vi "Read data.vi"(7 "Command":T1, 8 "error in":errorcluster, 11 "file path":path) -> (0 "error out":errorcluster, 2 "Zone Setup Array":cluster{string, dbl}[](array[cluster]))   [LabVIEW 2013]
doc: "This SubVI is used to\n-Initialize the file path and stores it in shift register.\n-Reads the data from the stored file path.\n-Empty the file path."
uses:
  Controls/Read States.ctl
  <vilib>/Utility/file.llb/Read From Spreadsheet File (string).vi
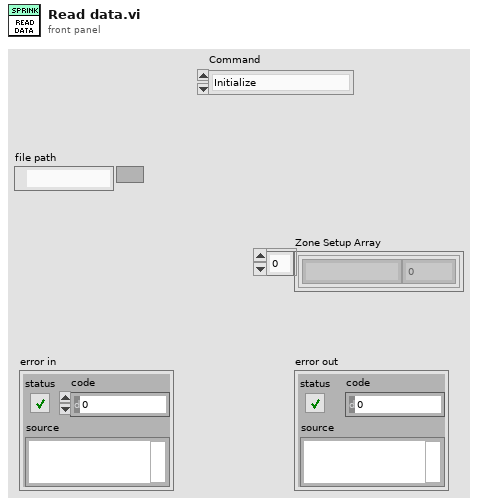
[diagram p1: front panel]
types:
  T1 = typedef "Read States.ctl" = enum16{"Initialize ", "Read", "Stop"}
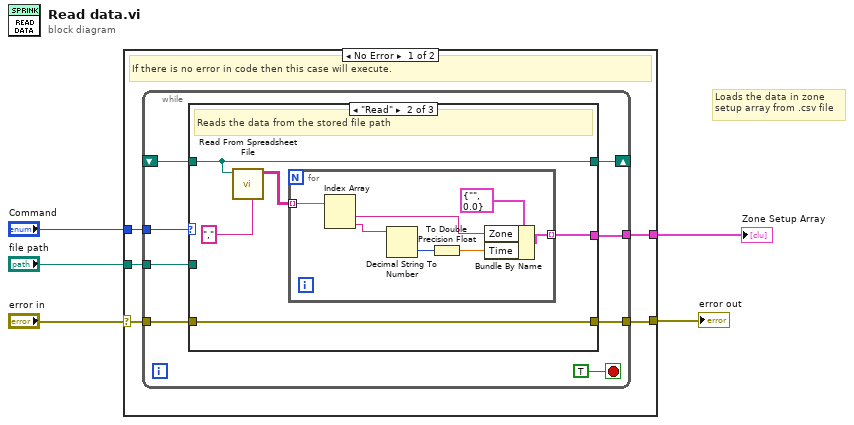
[diagram p0: block diagram]
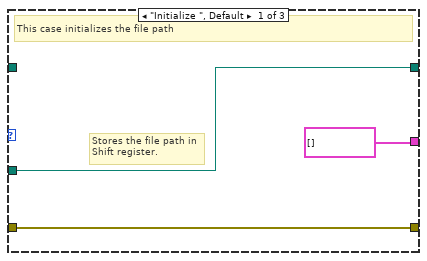
[diagram p2: hidden frame]
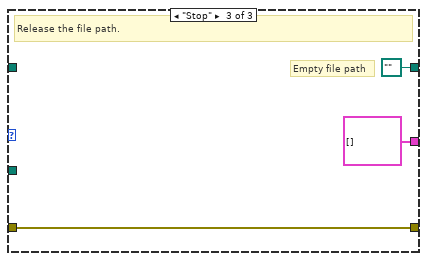
[diagram p3: hidden frame]
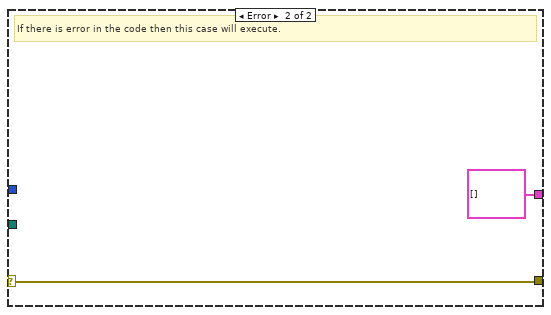
[diagram p4: hidden frame]
diagram:
  # "Loads the data in zone \nsetup array from .csv file"
  n1 = case shown="No Error" "error in" {
    selector: "error in" -> [w6 w38]
    tunnel: "Command" -> [w10 _]
    tunnel: "file path" -> [w9 _]
    tunnel: [w8 cluster{"Zone":string, "Time":dbl}[] [] ("Array")] -> w1
    tunnel: [w7 w38] -> w5
    frame No Error {
      # "If there is no error in code then this case will execute."
      n2 = while {
        tunnel: w10 -> [w17]
        tunnel: w9 -> [w16]
        shift-right: [w15] -> _
        shift-left: _ -> [w14]
        tunnel: [w13] -> w8
        tunnel: [w12] -> w7
        tunnel: w6 -> [w11]
        stop <- TRUE stop-if-true
        n3 = case shown="\"Read\"" w17 {
          tunnel: w16 -> [w21 _ _]
          tunnel: [w21 w25 path "" ("file path")] -> w15
          tunnel: w14 -> [_ w25 _]
          tunnel: [cluster{string, dbl}[] [] ("Array") w22 cluster{"Zone":string, "Time":dbl}[] [] ("Array")] -> w13
          tunnel: [w20 w24 w35] -> w12
          tunnel: w11 -> [w20 w24 w35]
          frame "Initialize ", Default {
            # "Stores the file path in\nShift register."
            # "This case initializes the file path"
          }
          frame "Read" {
            # "Reads the data from the stored file path"
            n4 = call-poly <vilib>:"Read From Spreadsheet File.vi"("delimiter (\\t)"="," ("delimiter (\\t)"), "file path (dialog if empty)"=w25) -> ("all rows"=w23:string[][])  [unwired: 5 in, 4 out]
            n5 = for {
              tunnel: w23 -> [w33] mode=indexing
              tunnel: [w32] -> w22 mode=indexing
              n6 = Index Array(array=w33) -> (element #1=w30:string, element #2=w29:string)  [unwired: 2 in]
              n7 = Decimal String To Number(string=w29) -> (number=w28:i32)  [unwired: 2 in, 1 out]
              n8 = To Double Precision Float(number=w28) -> (double precision float=w27:dbl)
              n9 = Bundle By Name(cluster=cluster{"Zone":string, "Time":dbl} {"Zone"="", "Time"=0.0}, "Zone"=w30, "Time"=w27) -> (w32:cluster{"Zone":string, "Time":dbl})
            }
          }
          frame "Stop" {
            # "Empty file path"
            # "Release the file path."
          }
        }
      }
    }
    frame Error {
      # "If there is error in the code then this case will execute."
    }
  }
  "error out" <- w5
  "Zone Setup Array" <- w1
